vi "get_bounding_box.vi"(8 "error in (no error)":errorcluster, 11 "RoiGeneric in":refnum<class "RoiGeneric.lvclass">) -> (0 "error out":errorcluster, 2 "Box.lvclass":refnum<class "Box.lvclass">, 3 "RoiGeneric out":refnum<class "RoiGeneric.lvclass">)   [LabVIEW 2010, in "RoiGeneric.lvclass"]
uses:
  RoiGeneric.lvclass
  common/classes/Box/Box/Box.lvclass
  RoiGeneric.lvclass/RoiGeneric.ctl
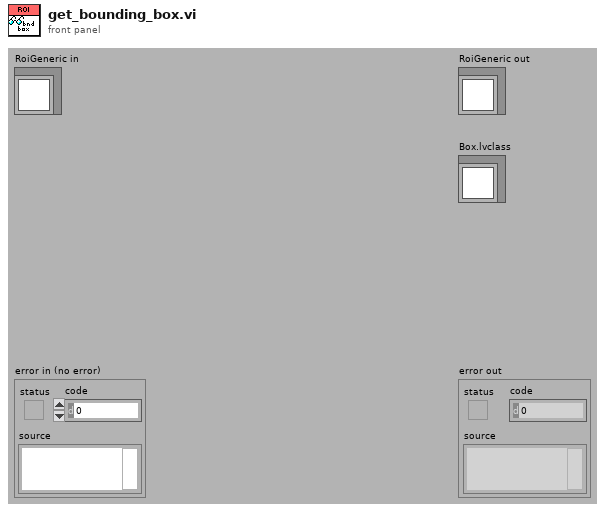
[diagram p1: front panel]
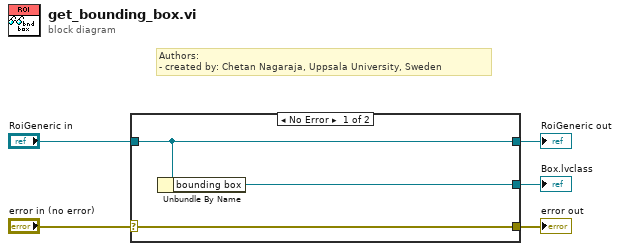
[diagram p0: block diagram]
diagram:
  # "Authors: \n- created by: Chetan Nagaraja, Uppsala University, Sweden"
  n1 = case shown="No Error" "error in (no error)" {
    selector: "error in (no error)" -> [w8 w9]
    tunnel: [w8 w9] -> w4
    tunnel: [w7 w10] -> w2
    tunnel: "RoiGeneric in" -> [w7 w10]
    tunnel: [w6 _] -> w1
    frame No Error {
      n2 = Unbundle By Name(w7) -> ("bounding box"=w6:refnum<class "Box.lvclass">)
    }
    frame Error {
    }
  }
  "error out" <- w4
  "RoiGeneric out" <- w2
  "Box.lvclass" <- w1
